vi "WPI_AnalogChannelERRSetOnUnallocatedChannel.vi"() -> (0 "error out":errorcluster)   [LabVIEW 2017]
doc: "This software is licensed. Open the labview\\readme\\WPI Robotics Library Open Source License.txt file for more information."
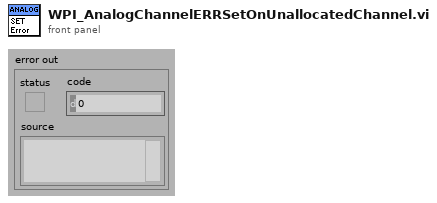
[diagram p1: front panel]
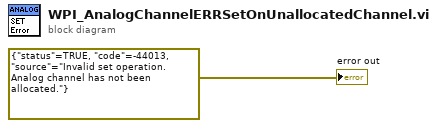
[diagram p0: block diagram]
diagram:
  "error out" <- errorcluster {"status"=TRUE, "code"=-44013, "source"="Invalid set operation. Analog channel has not been allocated."} ("ERRAllocAnInvalidCounterIdx")
